vi "Get Project References.vi"(8 "error in":errorcluster, 10 "Target Selection":string, 11 "Project in":refnum<vi>) -> (0 "error out":errorcluster, 3 "Project":refnum<class "Project.lvclass">)   [LabVIEW 2019, in "Panther Dashboard.lvlib" / "Project.lvclass"]
uses:
  Project.lvclass
  Project.lvclass/Project.ctl
  Write Project Description.vi
  Write Project Ref.vi
  Write Project Name.vi
  Write Target Name.vi
  Write Target Ref.vi
  Write Target App Ins Ref.vi
  Write Main App Inst Ref.vi
  Write Project Path.vi
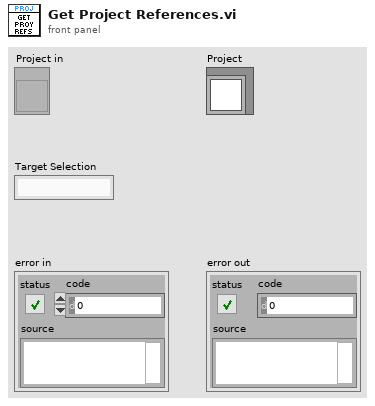
[diagram p1: front panel]
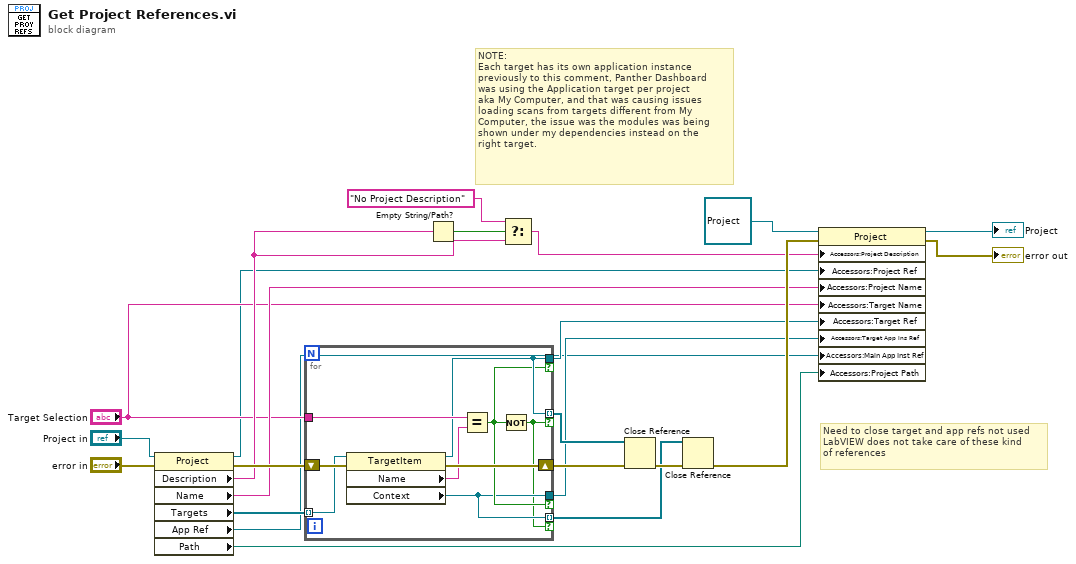
[diagram p0: block diagram]
diagram:
  # "NOTE:\nEach target has its own application instance\npreviously to this comment, Panther Dashboard\nwas using the Application target per project \naka My Computer, and that was causing issues \nloading scans from targets different from My\nComputer, the issue was the modules was being\nshown under my dependencies instead on the\nright target."
  # "Need to close target and app refs not used\nLabVIEW does not take care of these kind\nof references"
  n1 = property class="Project"(reference="Project in", error in="error in") -> (reference out=w3:refnum<vi>, error out=w21:errorcluster, "Description"=w12:string, "Name"=w9:string, "Targets"=w14:refnum<vi>[], "App Ref"=w5:refnum<vi>, "Path"=w1:path)
  n2 = for {
    tunnel: w14 -> [w30] mode=indexing
    tunnel: "Target Selection" -> [w28]
    tunnel: [w27] -> w7 if=w26
    tunnel: [w27] -> w17 mode=indexing if=w24
    shift-right: [w31] -> w20
    shift-left: w21 -> [w32]
    tunnel: [w25] -> w6 if=w26
    tunnel: [w25] -> w11 mode=indexing if=w24
    n3 = property class="TargetItem"(reference=w30, error in=w32) -> (reference out=w27:refnum<vi>, error out=w31:errorcluster, "Name"=w29:string, "Context"=w25:refnum<vi>)
    n4 = Equal?(x=w28, y=w29) -> (x = y?=w26:bool)
    n5 = Not(x=w26) -> (.not. x?=w24:bool)
  }
  n6 = Empty String/Path?(string/path=w12) -> (empty?=w15:bool)
  n7 = Select(t="No Project Description", s=w15, f=w12) -> (s? t:f=w2:string)
  n8 = Close Reference(reference=w17, error in (no error)=w20) -> (error out=w22:errorcluster)
  n9 = Close Reference(reference=w11, error in (no error)=w22) -> (error out=w19:errorcluster)
  n10 = property class="Project"(reference=refnum<class "Project.lvclass"> refnum ("Project.lvclass"), error in=w19, "Accessors:Project Description"=w2, "Accessors:Project Ref"=w3, "Accessors:Project Name"=w9, "Accessors:Target Name"="Target Selection", "Accessors:Target Ref"=w7, "Accessors:Target App Ins Ref"=w6, "Accessors:Main App Inst Ref"=w5, "Accessors:Project Path"=w1) -> (reference out=→"Project":refnum<class "Project.lvclass">, error out=→"error out":errorcluster)
